vi "DPIDs.Compile.vi"(8 "error in (no error)":errorcluster, 10 "PIDs":T3[](array[typedef]) {"Signals"."Byte Order" items=["Little Endian", "Big Endian"]; "Signals"."Data Type" items=["Signed", "Unsigned", "IEEE Float"]}, 11 "DPIDs":T1[](array[typedef])) -> (0 "error out":errorcluster, 3 "Lookup Table":variant)   [LabVIEW 2024, in "Diagnostics Addon System Explorer.lvlib"]
uses:
  Diagnostics Addon System Explorer.lvlib
  Addon Shared/Types/Frame.Compile.ctl
  Addon Shared/Types/Type.ctl
  Addon Shared/Types/Signal.ctl
  Addon Shared/Types/DPID.ctl
  Addon Shared/Types/DPID.Rate.ctl
  Addon Shared/Types/DPID.Lookup.Info.ctl
  Addon Shared/Types/DPID.Lookup.Info.PID.ctl
  Addon Shared/Diagnostics Addon Shared.lvlib
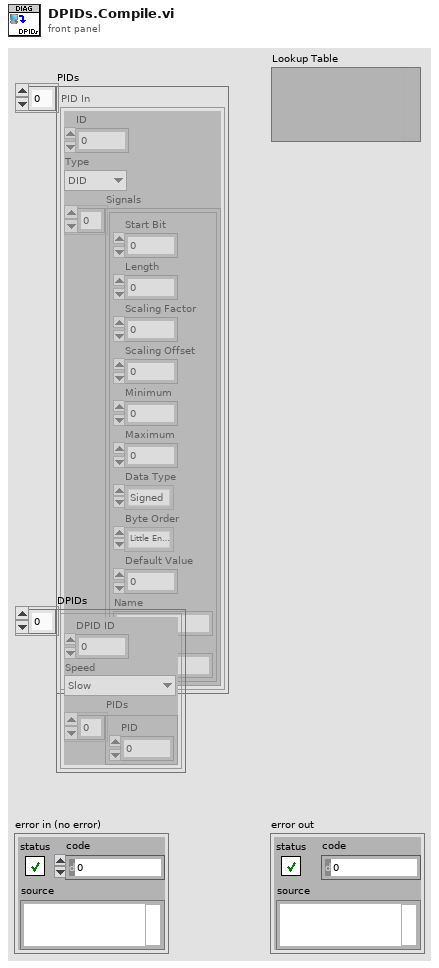
[diagram p1: front panel]
types:
  T1 = typedef "Diagnostics Addon Shared.lvlib/DPID.ctl" = cluster{"DPID ID":u8, "Speed":T2, "PIDs":u16[]}
  T2 = typedef "Diagnostics Addon Shared.lvlib/DPID.Rate.ctl" = enum16{"Slow", "Medium", "Fast"}
  T3 = typedef "Diagnostics Addon Shared.lvlib/Frame.Compile.ctl" = cluster{"ID":u32, "Type":T4, "Signals":T5[]}
  T4 = typedef "Diagnostics Addon Shared.lvlib/Type.ctl" = enum16{"DID", "CDID", "PID", "CPID", "Read Memory", "Write Memory", "IO Control", "Routine Start", "Routine Request", "Routine Stop", "User Defined", "DTC Control", "Clear DTCs", "Read DTCs", "Start DTCs", "DTC Change Count", "Tester Present", "Unlock ECU", "Reset ECU", "Diag Session Control", "Communication Control", "DPID Control", "Poll Control", "Diag Comm Port Control"}
  T5 = typedef "Diagnostics Addon Shared.lvlib/Signal.ctl" = cluster{"Start Bit":u32, "Length":u32, "Scaling Factor":dbl, "Scaling Offset":dbl, "Minimum":dbl, "Maximum":dbl, "Data Type":u32, "Byte Order":u32, "Default Value":dbl, "Name":string, "Units":string}
  T6 = typedef "Diagnostics Addon Shared.lvlib/DPID.Lookup.Info.ctl" = cluster{"PID Info":T7}
  T7 = typedef "Diagnostics Addon Shared.lvlib/DPID.Lookup.Info.PID.ctl" = cluster{"PID":u16, "Frame Length":u8}
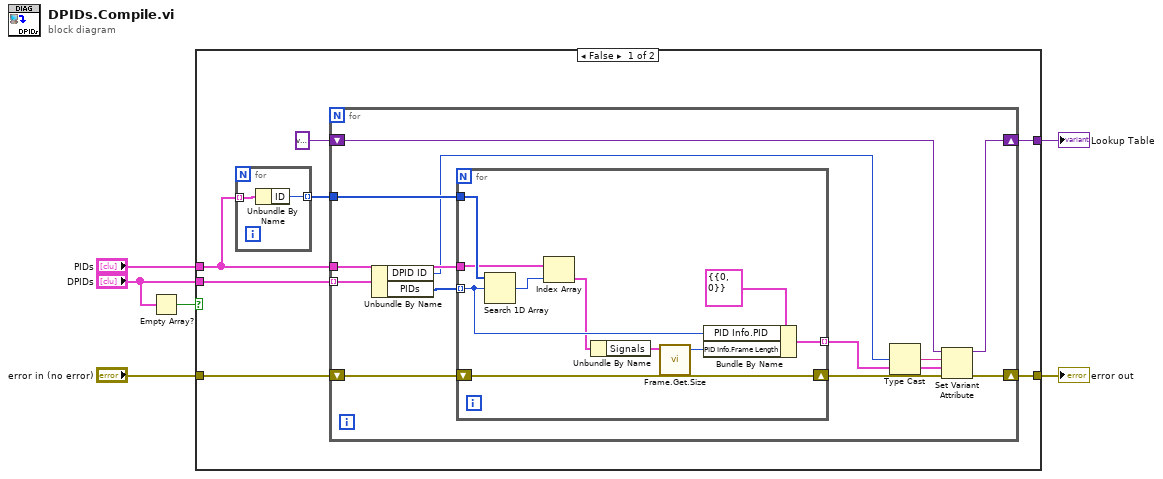
[diagram p0: block diagram]
diagram:
  n1 = Empty Array?(array="DPIDs") -> (empty?=w1:bool)
  n2 = case shown="False" w1 {
    tunnel: "error in (no error)" -> [w12 w38]
    tunnel: [w11 _] -> w5
    tunnel: "PIDs" -> [w10 _]
    tunnel: "DPIDs" -> [w8 _]
    tunnel: [w7 w38] -> w3
    frame False {
      n3 = for {
        tunnel: w10 -> [w15] mode=indexing
        tunnel: [w14] -> w9 mode=indexing
        n4 = Unbundle By Name(w15) -> ("ID"=w14:u32)
      }
      n5 = for {
        tunnel: w8 -> [w27] mode=indexing
        tunnel: w9 -> [w26]
        tunnel: w10 -> [w24]
        shift-right: [w17] -> w11
        shift-left: variant -> [w23]
        shift-right: [w18] -> w7
        shift-left: w12 -> [w21]
        n6 = Unbundle By Name(w27) -> ("DPID ID"=w22:u8, "PIDs"=w25:u16[])
        n7 = for {
          tunnel: w26 -> [w37]
          tunnel: w25 -> [w33] mode=indexing
          tunnel: w24 -> [w36]
          shift-right: [w34] -> w20
          shift-left: w21 -> [w34]
          tunnel: [w32] -> w16 mode=indexing
          n8 = Search 1D Array(1D array=w37, element=w33) -> (index of element=w35:i32)  [unwired: 1 in]
          n9 = Index Array(array=w36, index=w35) -> (element=w30:T3)
          n10 = Unbundle By Name(w30) -> ("Signals"=w29:T5[])
          n11 = call "Frame.Get.Size.vi"("Parameters"=w29) -> ("Bytes"=w28:u32)  [unwired: 10 in]
          n12 = Bundle By Name(cluster=T6 {"PID Info"={"PID"=0, "Frame Length"=0}} ("Cluster"), "PID Info.PID"=w33, "PID Info.Frame Length"=w28) -> (w32:T6)
        }
        n13 = Type Cast(x=w22) -> (*(type *) &x=w19:string)  [unwired: 1 in]
        n14 = Set Variant Attribute(Variant=w23, name=w19, value=w16, error in=w20) -> (Variant out=w17:variant, error out=w18:errorcluster)  [unwired: 1 out]
      }
    }
    frame True {
    }
  }
  "error out" <- w3
  "Lookup Table" <- w5
